vi "a2.vi"(4 "error in":errorcluster, 7 "Image In":T1) -> (0 "error out":errorcluster, 1 "Calibrated Results (Caliper 2)":sgl[][](array[numeric]) format="%.2f", 2 "Calibrated Results (Caliper 1)":sgl[][](array[numeric]) format="%.2f", 3 "Image Out":T1, 5 "Caliper Results (Caliper 1)":sgl[][](array[numeric]) format="%.2f", 6 "Caliper Results (Caliper 2)":sgl[][](array[numeric]) format="%.2f")   [LabVIEW 2015]
uses:
  <vilib>/vision/Image Controls.llb/IMAQ Image.ctl
  <vilib>/vision/NI_Vision_Development_Module.lvlib
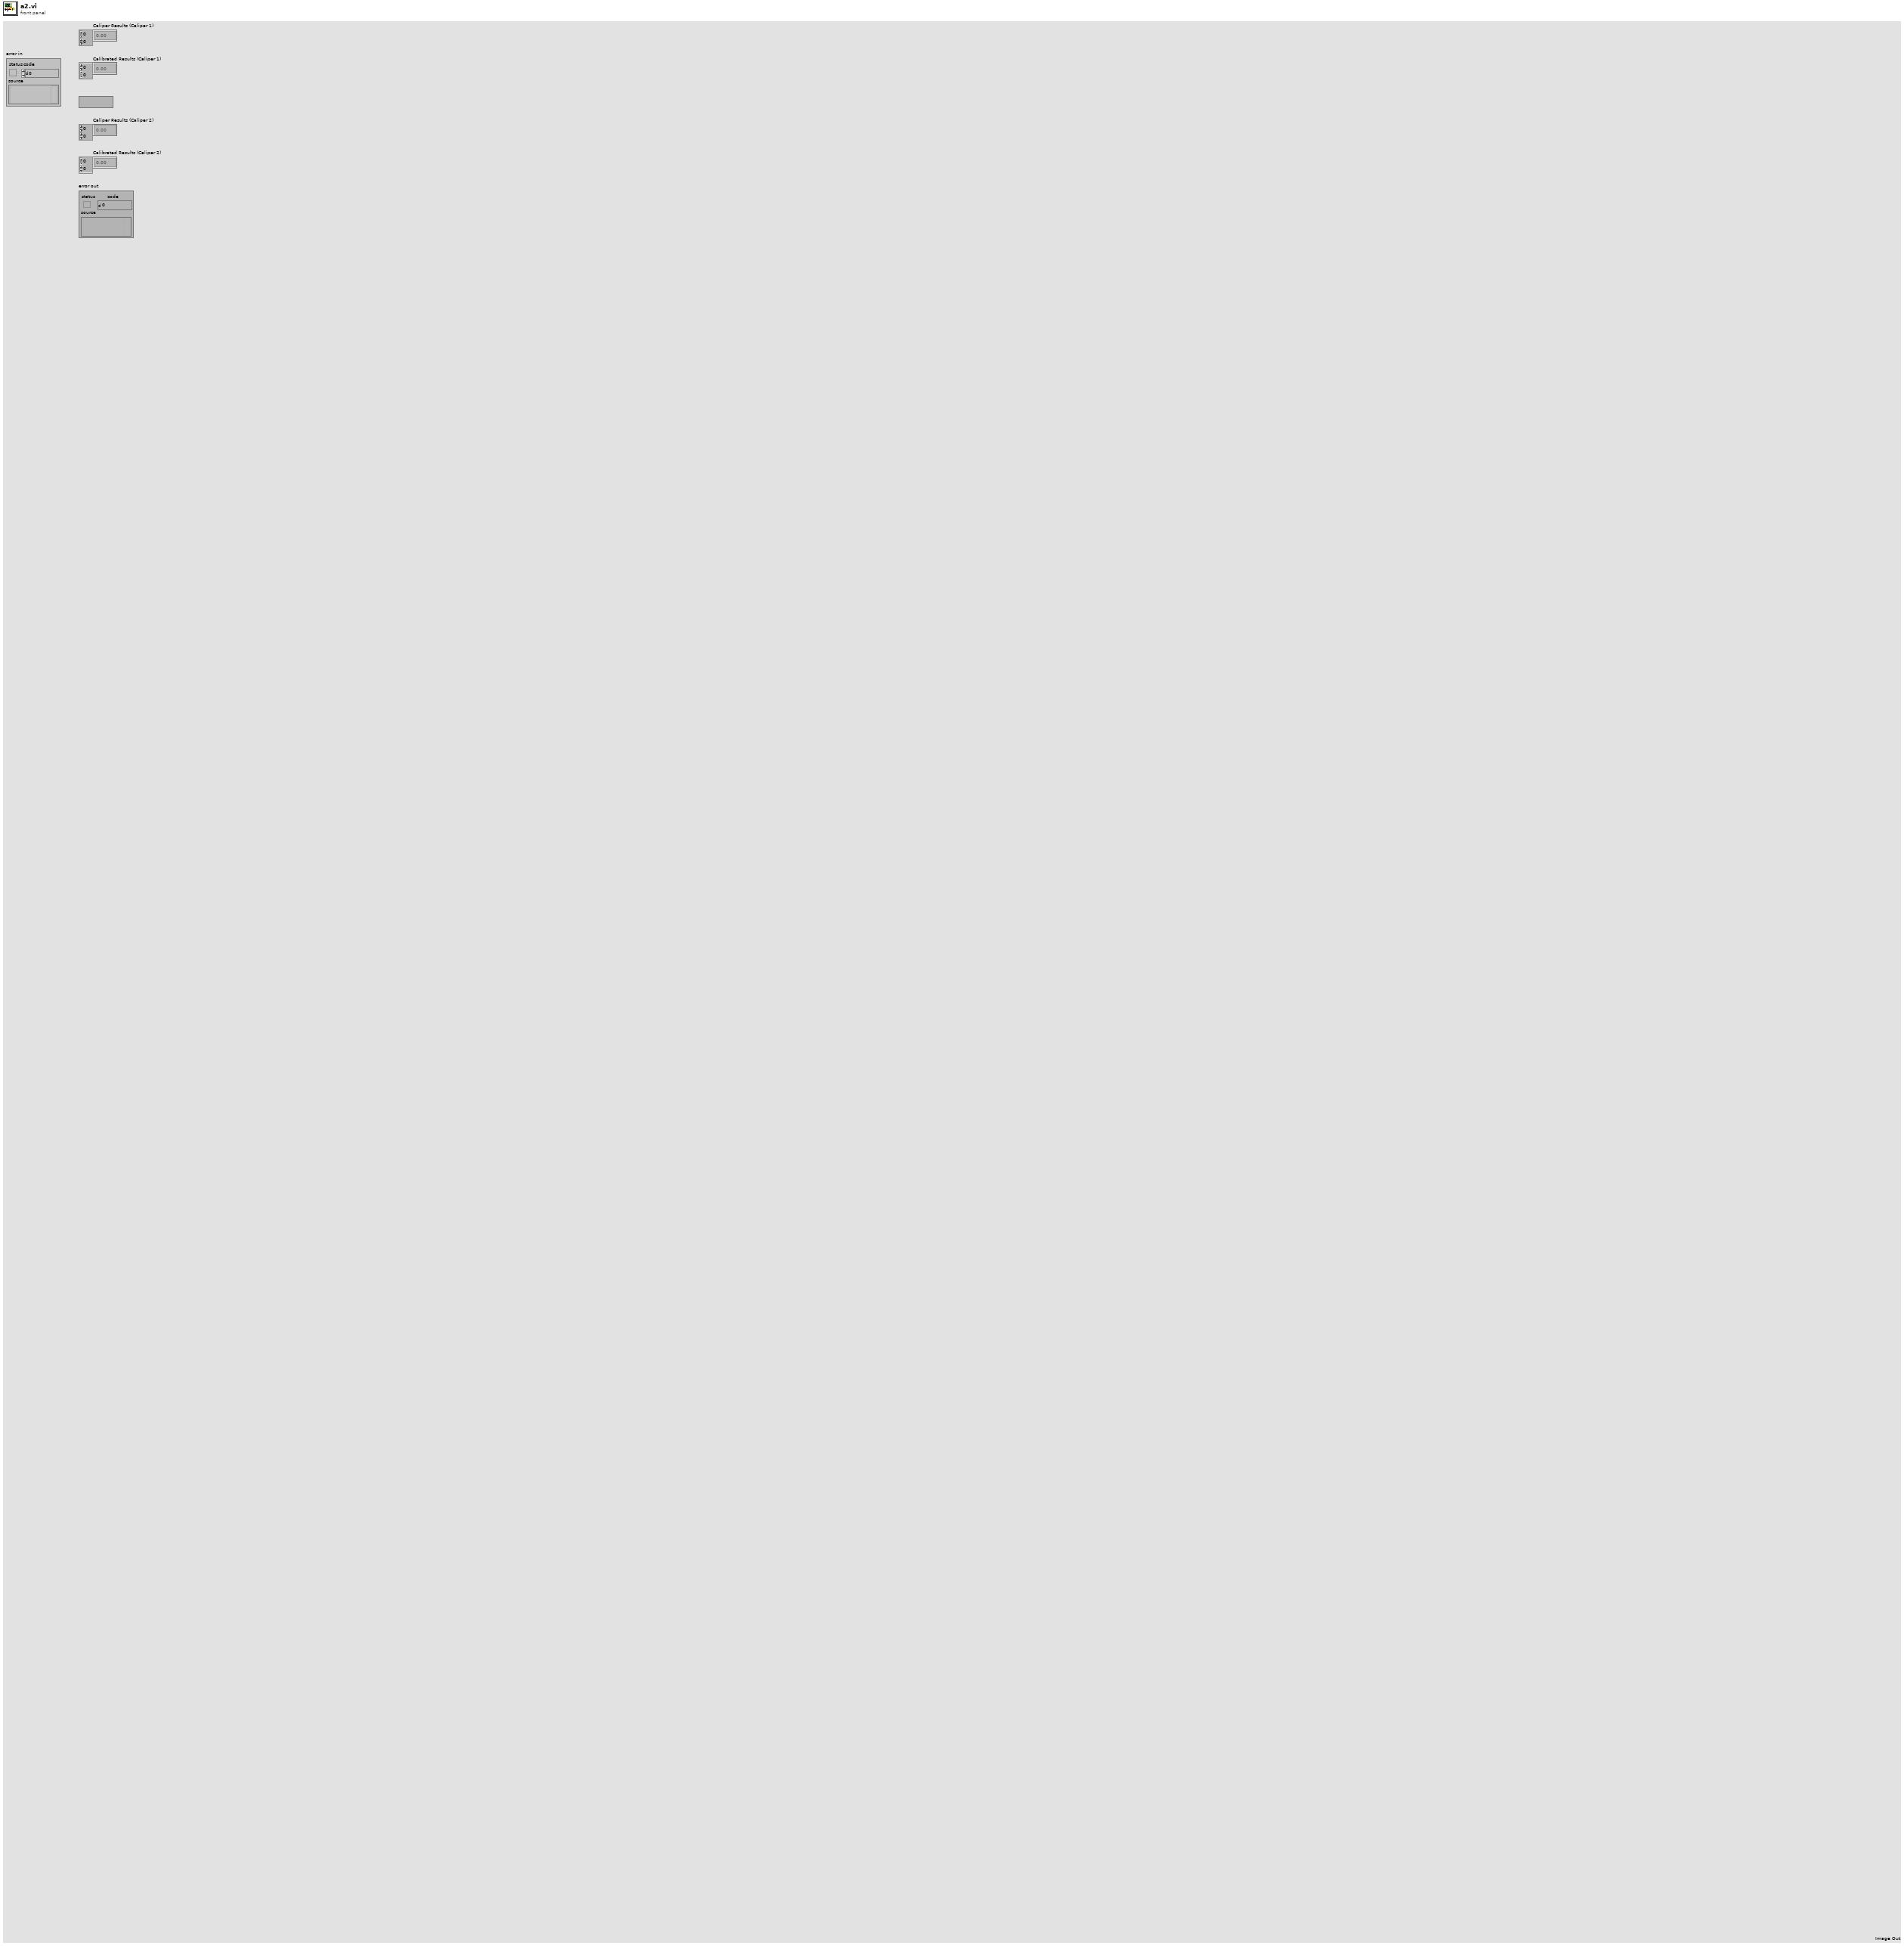
[diagram p1: front panel]
types:
  T1 = typedef "IMAQ Image.ctl" = refnum<image>
  T2 = cluster{"Feature":u32, "Points IDs":cluster{"GUID":string, "Index":i32}[]}[]
  T3 = cluster{"Edge Polarity":u32, "Kernel Size":u32, "Width":u32, "Minimum Edge Strength":sgl, "Interpolation Type":enum32{"Zero Order", "Bilinear", "Quadratic", "Cubic", "Bilinear Fixed"}, "Data Processing Method":enum32{"Average", "Median"}}
  T4 = enum16{"Get First Edge", "Get First + Last Edge", "Get All Edges", "Get Best Edge"}
  T5 = cluster{"Global Rectangle":i32[], "Contours":cluster{"ID":enum32{"External", "Internal"}, "Type":u32, "Coordinates":i32[]}[]}
  T6 = cluster{"Sigma":sgl, "HThresh":sgl, "LThres":sgl, "WindowSize":i32}
  T7 = cluster{"Brightness":sgl, "Contrast":sgl, "Gamma":sgl}
  T8 = typedef "Edge New.ctl" = cluster{"Location (Pixel)":cluster{"X":sgl, "Y":sgl}, "Location (Real-World)":cluster{"X":sgl, "Y":sgl}, "Distance (Pixel)":dbl, "Distance (Real-World)":dbl, "Strength":dbl, "Noise":dbl, "Rising?":bool}
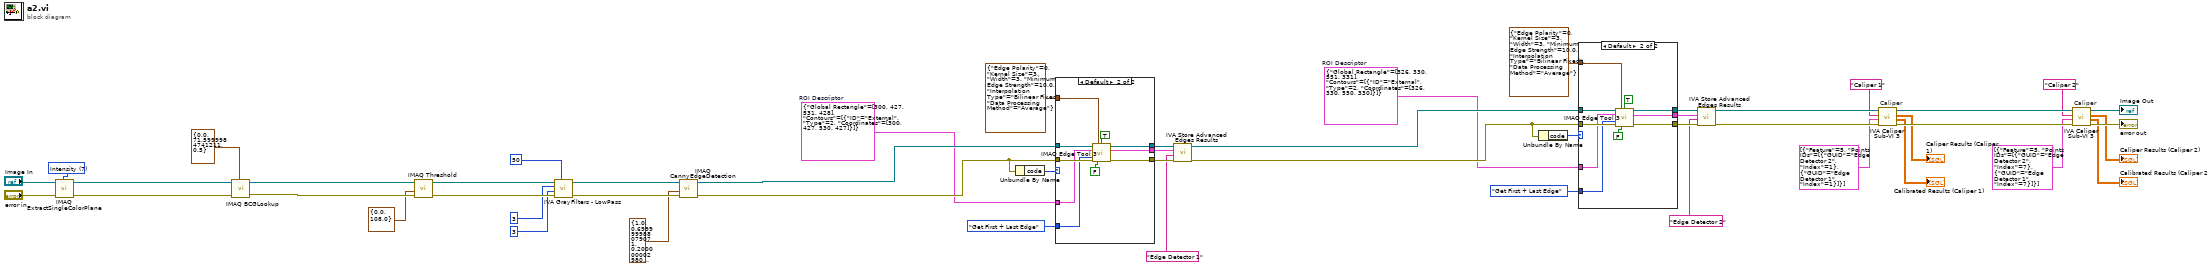
[diagram p0: block diagram]
diagram:
  w15 = T5 {"Global Rectangle"=[326, 330, 551, 331], "Contours"=[{"ID"=enum."External", "Type"=2, "Coordinates"=[326, 330, 550, 330]}]}  # ROI Descriptor
  w25 = T5 {"Global Rectangle"=[300, 427, 531, 428], "Contours"=[{"ID"=enum."External", "Type"=2, "Coordinates"=[300, 427, 530, 427]}]}  # ROI Descriptor
  w51 = 7 items=["Red", "Green", "Blue", "Hue", "Saturation", "Luminance", "Value", "Intensity"] ("Color Plane")
  # "Caliper"
  # "Caliper"
  n1 = call "IMAQ ExtractSingleColorPlane"("Color Plane"=w51, "error in (no error)"="error in", "Image Src"="Image In") -> ("error out"=w48:errorcluster, "Image Dst Out"=w46:T1)  [unwired: 1 in, 6 out]
  n2 = call "IMAQ BCGLookup"("Image Src"=w46, "BCG Values"=T7 {"Brightness"=0.0, "Contrast"=71.6, "Gamma"=0.5}, "error in (no error)"=w48) -> ("Image Dst Out"=w43:T1, "error out"=w47:errorcluster)  [unwired: 2 in, 2 out]
  n3 = call "IMAQ Threshold"("error in (no error)"=w47, "Range"=cluster{"Lower value":sgl, "Upper value":sgl} {"Lower value"=0.0, "Upper value"=108.0}, "Image Src"=w43) -> ("error out"=w42:errorcluster, "Image Dst Out"=w41:T1)  [unwired: 3 in, 4 out]
  n4 = call <vilib>:"IVA GrayFilters - LowPass.vi"("Tolerance"=50, "error in"=w42, "Filter size Y"=3, "Filter size X"=3, "Image In"=w41) -> ("error out"=w40:errorcluster, "Image Out"=w36:T1)  [unwired: 5 out]
  n5 = call "IMAQ CannyEdgeDetection"("Image Src"=w36, "Filter Parameters"=T6 {"Sigma"=1.0, "HThresh"=0.7, "LThres"=0.2, "WindowSize"=9}, "error in (no error)"=w40) -> ("Image Dst Out"=w33:T1, "error out"=w35:errorcluster)  [unwired: 1 in, 4 out]
  n6 = Unbundle By Name(w35) -> ("code"=w24:i32)
  n7 = case shown="Default" w24 {
    tunnel: w35 -> [_ w62]
    tunnel: w33 -> [w52 w61]
    tunnel: T4."Get First + Last Edge" ("Process") -> [_ w60]
    tunnel: T3 {"Edge Polarity"=0, "Kernel Size"=3, "Width"=3, "Minimum Edge Strength"=10.0, "Interpolation Type"=enum."Bilinear Fixed", "Data Processing Method"=enum."Average"} ("Edge Options") -> [_ w59]
    tunnel: [_ w58] -> w30
    tunnel: [w52 w57] -> w28
    tunnel: [_ w56] -> w27
    tunnel: w25 -> [_ w55]
    frame -1074396199, -1074396198 {
    }
    frame Default {
      n8 = call "IMAQ Edge Tool 3"("Image"=w61, "Edge Options"=w59, "Optimized Mode"=TRUE, "ROI Descriptor"=w55, "Process"=w60, "error in (no error)"=w62, "Reverse Direction"=FALSE) -> ("Image (duplicate)"=w57:T1, "Edge Information"=w56:T8[], "error out"=w58:errorcluster)  [unwired: 6 out]
    }
  }
  n9 = call <vilib>:"IVA Store Advanced Edges Results.vi"("error in (no error)"=w30, "Step Name"="Edge Detector 1", "Edge Information"=w27, "Image in"=w28) -> ("error out"=w29:errorcluster, "Image dup"=w23:T1)  [unwired: 6 out]
  n10 = Unbundle By Name(w29) -> ("code"=w14:i32)
  n11 = case shown="Default" w14 {
    tunnel: w29 -> [_ w73]
    tunnel: w23 -> [w63 w72]
    tunnel: T4."Get First + Last Edge" ("Process") -> [_ w71]
    tunnel: T3 {"Edge Polarity"=0, "Kernel Size"=3, "Width"=3, "Minimum Edge Strength"=10.0, "Interpolation Type"=enum."Bilinear Fixed", "Data Processing Method"=enum."Average"} ("Edge Options") -> [_ w70]
    tunnel: [_ w69] -> w20
    tunnel: [w63 w68] -> w18
    tunnel: [_ w67] -> w17
    tunnel: w15 -> [_ w66]
    frame -1074396199, -1074396198 {
    }
    frame Default {
      n12 = call "IMAQ Edge Tool 3"("Image"=w72, "Edge Options"=w70, "Optimized Mode"=TRUE, "ROI Descriptor"=w66, "Process"=w71, "error in (no error)"=w73, "Reverse Direction"=FALSE) -> ("Image (duplicate)"=w68:T1, "Edge Information"=w67:T8[], "error out"=w69:errorcluster)  [unwired: 6 out]
    }
  }
  n13 = call <vilib>:"IVA Store Advanced Edges Results.vi"("error in (no error)"=w20, "Step Name"="Edge Detector 2", "Edge Information"=w17, "Image in"=w18) -> ("error out"=w19:errorcluster, "Image dup"=w13:T1)  [unwired: 6 out]
  n14 = call <vilib>:"IVA Caliper Sub-VI 3.vi"("error in"=w19, "Parameters"=T2 [{"Feature"=5, "Points IDs"=[{"GUID"="Edge Detector 2", "Index"=1}, {"GUID"="Edge Detector 1", "Index"=1}]}], "Step Name"="Caliper 1", "Image In"=w13) -> ("error out"=w12:errorcluster, "Results (Calibrated)"=→"Calibrated Results (Caliper 1)":sgl[][], "Results (Pixels)"=→"Caliper Results (Caliper 1)":sgl[][], "Image Out"=w7:T1)  [unwired: 1 in, 3 out]
  n15 = call <vilib>:"IVA Caliper Sub-VI 3.vi"("error in"=w12, "Parameters"=T2 [{"Feature"=5, "Points IDs"=[{"GUID"="Edge Detector 2", "Index"=7}, {"GUID"="Edge Detector 1", "Index"=7}]}], "Step Name"="Caliper 2", "Image In"=w7) -> ("error out"=→"error out":errorcluster, "Results (Calibrated)"=→"Calibrated Results (Caliper 2)":sgl[][], "Results (Pixels)"=→"Caliper Results (Caliper 2)":sgl[][], "Image Out"=→"Image Out":T1)  [unwired: 1 in, 3 out]
